vi "New Display GIC A.vi"(11 "GIC Input":T1={"     Use ?\nOff       On"=[FALSE, TRUE, FALSE, TRUE], "Mode:"=FALSE, "WP Data"="", "Hokuyo Port"="COM7", "Prop  Port"="COM6", "Compass Port"="", "GPS Port"="", "Num of WPs"=0, "WP Lats and Longs"={"WP Lats"=[], "WP Longs"=[]}, "Obst Lats and Longs"={"Obst Lats"=[], "Obst Longs"=[]}, "Parameters"=[], "GPS Data"=[], "Compass"=0.0, "LMS Vector"=[], "Vision Vector"=[], "Direction Cmd"=0.0, "Speed Cmd"=0.0, "WP Vector"=[], "WP Number"=0, "Extra"=0, "SW Map"=[], "Path Cluster"={"Path x node"=[], "Path y node"=[]}} {"Obst Lats and Longs"."Obst Longs" format="%#_8g"; "Obst Lats and Longs"."Obst Lats" format="%#_8g"}) -> (3 "Array":dbl[](array[numeric]))   [LabVIEW 2014]
panel:
  # "New Display GIC A"
  # "Output:"
  # "Input:"
  # "Robot Lat"
  # "Robot Long"
  # "Robot Heading"
  # "Robot Path Angle"
  # "Robot Speed"
  # "Angle to WP"
  # "Dist in Meters"
  # "WP Number"
  # "Next WP Lat"
  # "Next WP Long"
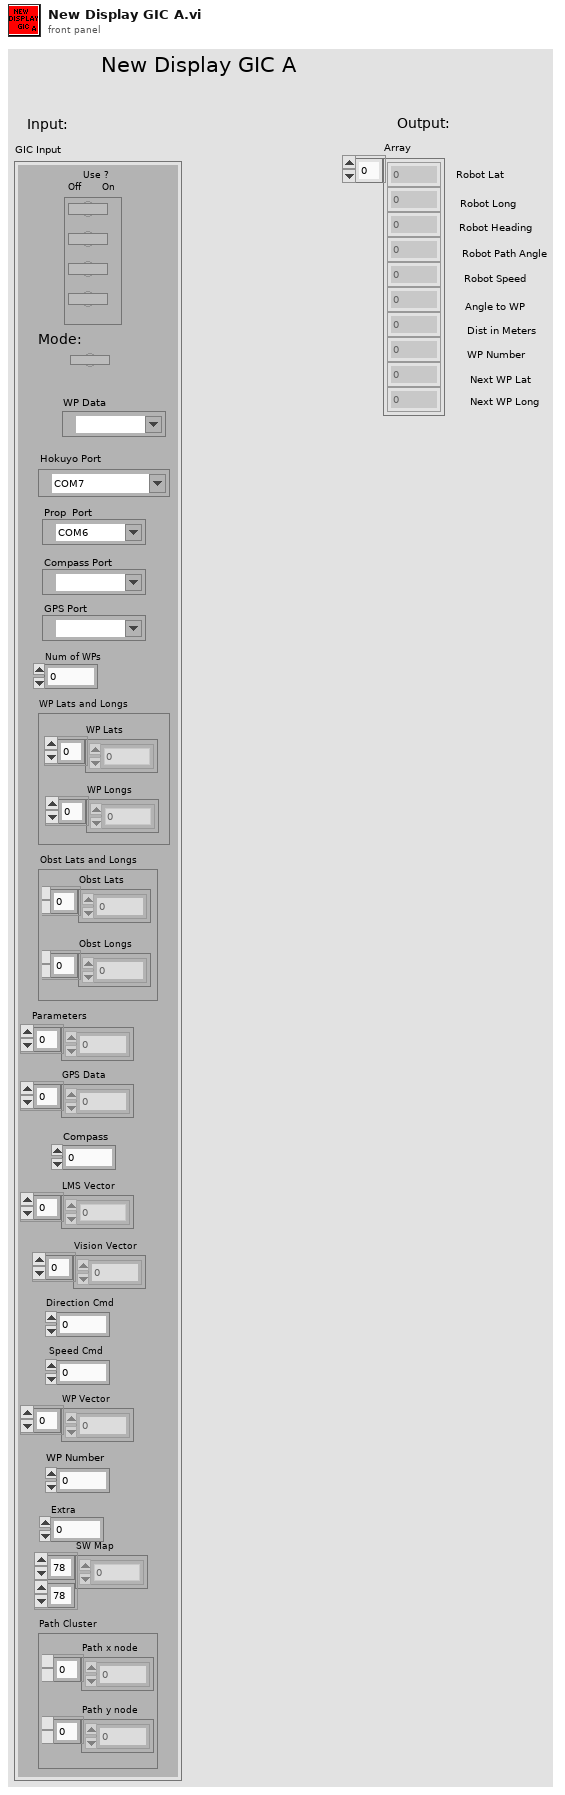
[diagram p1: front panel]
types:
  T1 = cluster{"     Use ?\nOff       On":bool[], "Mode:":bool, "WP Data":refnum<visa-resource-name>, "Hokuyo Port":refnum<visa-resource-name>, "Prop  Port":refnum<visa-resource-name>, "Compass Port":refnum<visa-resource-name>, "GPS Port":refnum<visa-resource-name>, "Num of WPs":i16, "WP Lats and Longs":cluster{"WP Lats":dbl[], "WP Longs":dbl[]}, "Obst Lats and Longs":cluster{"Obst Lats":dbl[], "Obst Longs":dbl[]}, "Parameters":dbl[], "GPS Data":dbl[], "Compass":dbl, "LMS Vector":dbl[], "Vision Vector":dbl[], "Direction Cmd":dbl, "Speed Cmd":dbl, "WP Vector":dbl[], "WP Number":i32, "Extra":i16, "SW Map":i32[][], "Path Cluster":cluster{"Path x node":dbl[], "Path y node":dbl[]}}
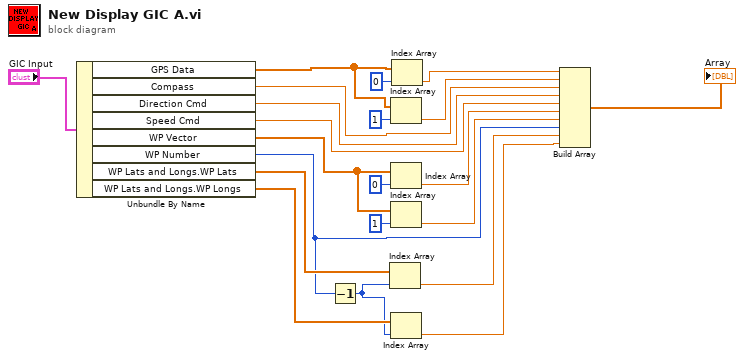
[diagram p0: block diagram]
diagram:
  n1 = Unbundle By Name("GIC Input") -> ("GPS Data"=w14:dbl[], "Compass"=w17:dbl, "Direction Cmd"=w13:dbl, "Speed Cmd"=w12:dbl, "WP Vector"=w10:dbl[], "WP Number"=w4:i32, "WP Lats and Longs.WP Lats"=w6:dbl[], "WP Lats and Longs.WP Longs"=w5:dbl[])
  n2 = Decrement(x=w4) -> (x-1=w3:i32)
  n3 = Index Array(array=w6, index=w3) -> (element=w2:dbl)
  n4 = Index Array(array=w14, index=1) -> (element=w18:dbl)
  n5 = Index Array(array=w10, index=0) -> (element=w8:dbl)
  n6 = Index Array(array=w10, index=1) -> (element=w7:dbl)
  n7 = Index Array(array=w5, index=w3) -> (element=w1:dbl)
  n8 = Index Array(array=w14, index=0) -> (element=w19:dbl)
  n9 = Build Array(w19, w18, w17, w13, w12, w8, w7, w4, w2, w1) -> (→"Array":dbl[])
